vi "Plate Tank 2.vi"() -> ()   [LabVIEW 2019]
uses:
  <vilib>/NI/Current Value Table/Type Defs/Single Tag.ctl
  <vilib>/NI/Current Value Table/Type Defs/Data Types.ctl
  <vilib>/Utility/sysdir.llb/System Directory Type.ctl
  <vilib>/NI/STM/TCP/Read Meta Data (TCP Ref).vi
  <vilib>/NI/STM/TCP/Get Connection Reference (TCP).vi
  <vilib>/NI/AMC/Read Termination Message.vi
  <vilib>/NI/AMC/Create Single Message.vi
  <vilib>/NI/AMC/Update Message Routing Info.vi
  <vilib>/NI/STM/TCP/Read Meta Data (TCP Clst).vi
  <vilib>/NI/AMC/Send Message.vi
  <vilib>/NI/AMC/Globals.vi
  <userlib>/_OpenG.lib/comparison/comparison.llb/I32 Changed__ogtk.vi
  <vilib>/NI/STM/TCP/Write Message (TCP).vi
  <vilib>/NI/AMC/AMC.lvlib
  <vilib>/NI/STM/NI STM.lvlib
  <vilib>/NI/Current Value Table/Current Value Table.lvlib
panel:
  in  "Settings Button":bool
  out "Loaded Recipe":string
  in  "Load A Recipe":bool
  in  "Save this Recipe":bool
  out "Right Time":dbl format="%.1f"
  out "Left Time":dbl format="%.1f"
  out "Total Amp*min R":dbl format="%.1f"
  out "Total Amp*min L":dbl format="%.1f"
  in  "Reverse Current Multiplier":dbl=3.0 min=0.1 max=100.0 step=0.01 format="%.2g"
  in  "Rectifer Settings":i32(listbox)
  in  "Tab Control 3":enum32{"Standard", "Eng"}(tab)
  out "Left Anode Amp-min":dbl(slide) scale=0.0..254.0
  out "Right Anode Amp-min":dbl(slide) scale=0.0..135.0
  out "Left Anode Actual Current":dbl(knob) scale=0.0..150.0
  out "Right Anode Actual Current":dbl(knob) scale=0.0..150.0
  out "Current Step":i32
  out "Output Voltage":cluster{dbl, dbl}(graph)
  in  "MO":string
  in  "Tab Control 2":enum32{"Plating Cell Status", "ENG"}(tab)
  out "Supply Flow":dbl(knob) scale=0.0..65.0 scale format="%#.2g"
  out "Suck Pump":bool
  out "Suck Pump Flow":dbl format="%#_4g"
  out "SuckPipe":bool
  out "Plating Cell Liquid Level":dbl(slide) scale=0.0..75.0
  out "Cell Temperature":dbl(slide) scale=0.0..60.0
  in  "Cell T Last Hr":bool
  in  "Tab Control":enum32{"Main Pump", "Suck Pump"}(tab)
  out "Amps":dbl format="%#.2g"
  out "Volts":dbl format="%#.1f"
  out "VFD T":dbl format="%#.2g"
  out "RPM":dbl format="%#.0f"
  out "Fault Code":dbl format="%#.2g"
  out "Freq":dbl format="%#.2g"
  out "SP1 Amps":dbl caption="Amps" format="%#.2g"
  out "SP1 Volts":dbl caption="Volts" format="%#.1g"
  out "SP1 RPM":dbl caption="RPM" format="%#.2g"
  out "SP1 VFD T":dbl caption="VFD T" format="%#.2g"
  out "SP1 Fault Code":dbl caption="Fault Code" format="%#.2g"
  out "SP1 Freq":dbl caption="Freq" format="%#.2g"
  out "Flow 1":dbl format="%#_4g"
  out "Flow 2":dbl format="%#_4g"
  out "Flow 3":dbl format="%#_4g"
  out "Flow 4":dbl format="%#_4g"
  out "Flow Controller":dbl(knob) scale=0.0..100.0
  out "E Stop":bool
  out "Run Enabled?":bool
  in  "Full Drain Plating Cell":bool
  out "Rack Motion":bool
  out "Right Eductor Motion":bool
  out "Left Eductor Motion":bool
  out "Right Output On":bool
  in  "Enable Rack Motion":bool
  in  "Rack RPM":dbl(knob) min=0.0 max=11.0 step=0.125 scale=0.0..11.0
  out "Left Output On":bool
  in  "Start Cycle":bool
  in  "Cancel Cycle":bool
  out "BasTankTee":bool
  out "SuckPipe 2":bool
  out "Main Pump":bool
  in  "Enable Eductor Motion":bool
  in  "Eductor RPM":dbl(knob) min=0.0 max=11.0 step=0.125 scale=0.0..11.0
  in  "Supply Pressure (kPa)":dbl(knob)=50.0 min=50.0 max=200.0 step=5.0 scale=50.0..200.0
  in  "Total Inflow (L/min)":dbl(knob)=40.0 min=25.0 max=50.0 step=1.0 scale=25.0..50.0
  in  "Suck Pump fraction of inflow":dbl(knob)=5.0 min=5.0 max=90.0 step=1.0 scale=0.0..90.0
  out "Sump Level":dbl(slide) scale=0.0..1000.0
  out "Supply Pressure":dbl(knob) scale=0.0..200.0
  in  "Enable Suck Pump":bool
  in  "Enable Plating Cell":bool
  in  "Machine":bool
  in  "Basement 4":bool
  in  "Dryer":bool
  in  "Rinse 4":bool
  in  "Rinse 3":bool
  in  "Rinse 2":bool
  in  "Basement 3":bool
  in  "Basement 2":bool
  in  "Basement 1":bool
  in  "Plater 6":bool
  in  "Plater 5":bool
  in  "Plater 4":bool
  in  "Plater 3":bool
  in  "Plater 2":bool
  in  "Plater 1":bool
  in  "Predip":bool
  in  "Rinse 1":bool
  in  "Cleaner":bool
  in  "Etch":bool
  out "status":string
  # "Module Selection"
  # "Rectifier Settings"
  # "Fluid Flow Control"
  # "Rectifier Control"
  # "Rectifier Output"
  # "Motion starts when rectifiers cycle"
  # "Note: RPM settings shared with tank 1"
  # "kPa"
  # "Output"
  # "cm"
  # "°C"
  # "cm"
  # "L/min"
  # "L/min"
  # "L/min"
  # "L/min"
  # "L/min"
  # "L/min"
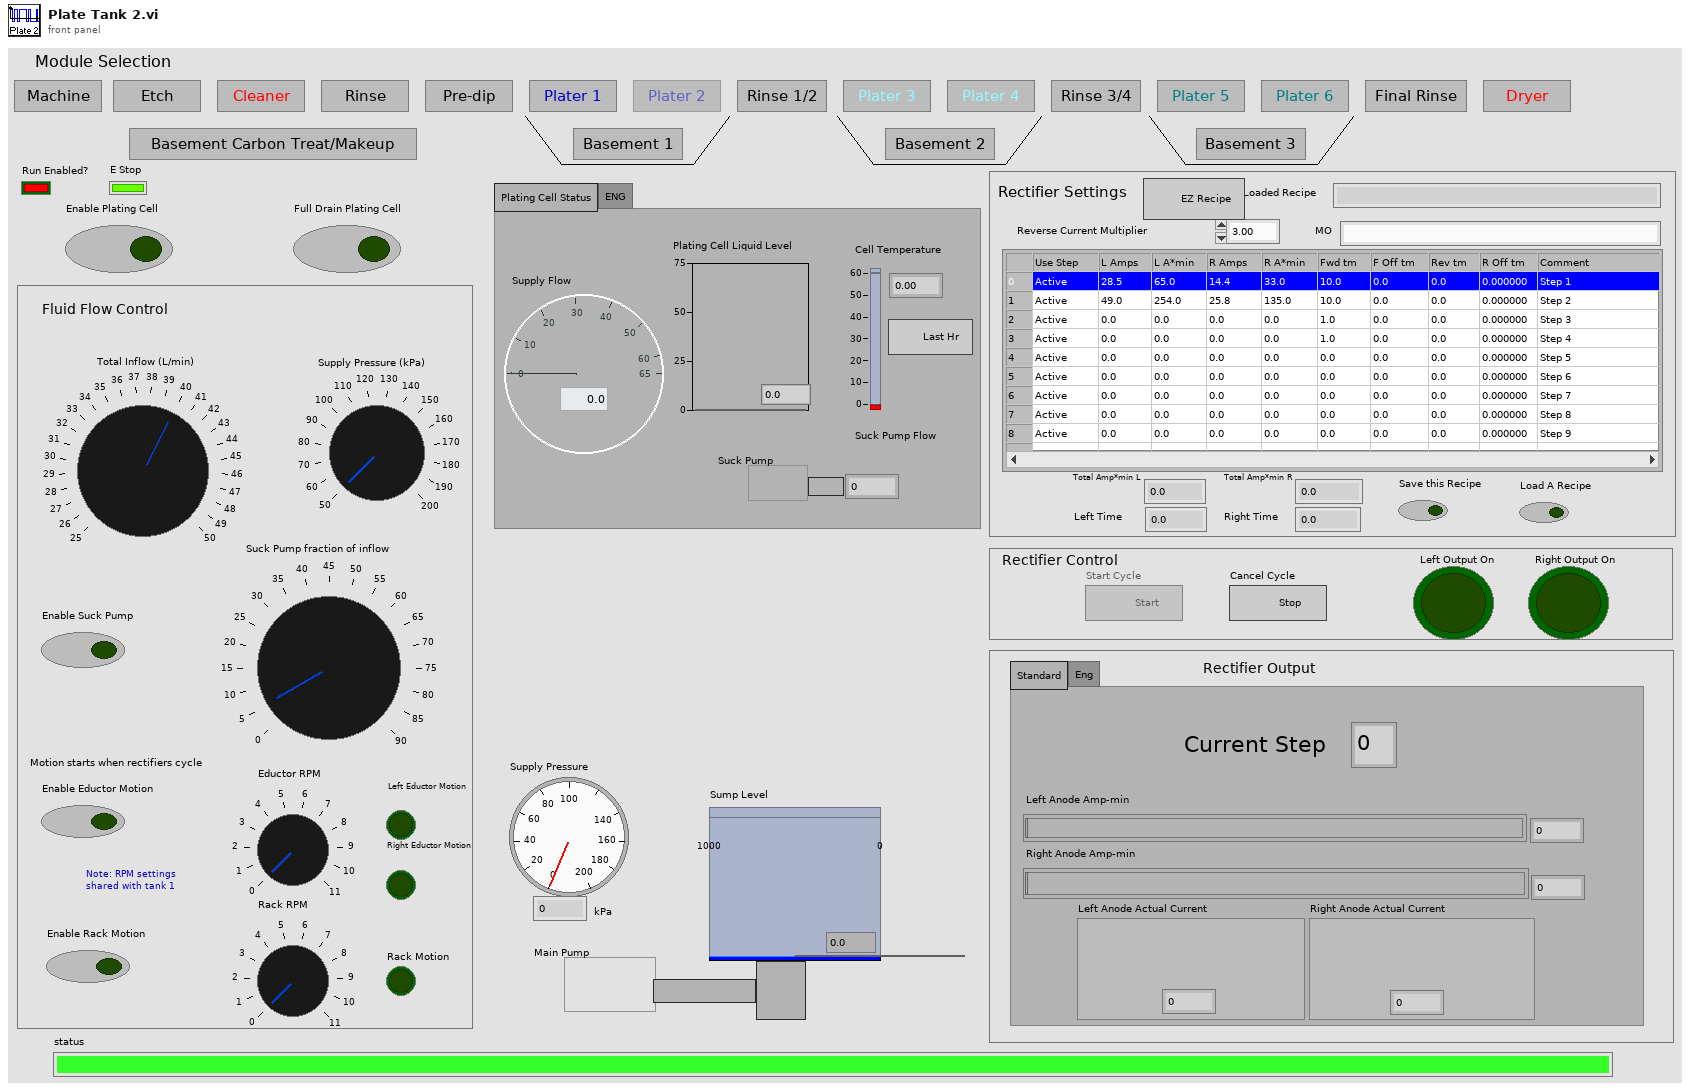
[diagram p1: front panel]
types:
  T1 = typedef "Current Value Table.lvlib/Single Tag.ctl" = cluster{"Data Type":T2, "Name":string, "Value":string, "Description":string}
  T2 = typedef "Current Value Table.lvlib/Data Types.ctl" = enum16{"Double", "Single", "I64", "I32", "I16", "I8", "U64", "U32", "U16", "U8", "String", "Boolean", "Array of U8", "Array of U16", "Array of U32", "Array of U64", "Array of I64", "Array of I32", "Array of I16", "Array of I8", "Array of Double", "Array of Single", "Array of Boolean", "Array of String"}
  T3 = typedef "NI STM.lvlib/TCP Connection Info.ctl" = cluster{"connection ID":refnum<k5>, "meta data":T4[]}
  T4 = typedef "NI STM.lvlib/MetaDataElement.ctl" = string
  T5 = typedef "AMC.lvlib/Message Queue.ctl" = refnum<queue>
  T6 = enum8{"Enabled", "Disabled", "Disabled and Grayed Out"}
  T7 = typedef "System Directory Type.ctl" = i32
  T8 = cluster{"Shift":bool, "Ctrl":bool, "Alt":bool, "Cmd":bool, "Opt":bool}
  T9 = typedef "LVPoint32TypeDef.ctl" = cluster{"Horizontal":i32, "Vertical":i32}
  T10 = typedef "LVRowAndColumnTypeDef.ctl" = cluster{"Row":i32, "Column":i32}
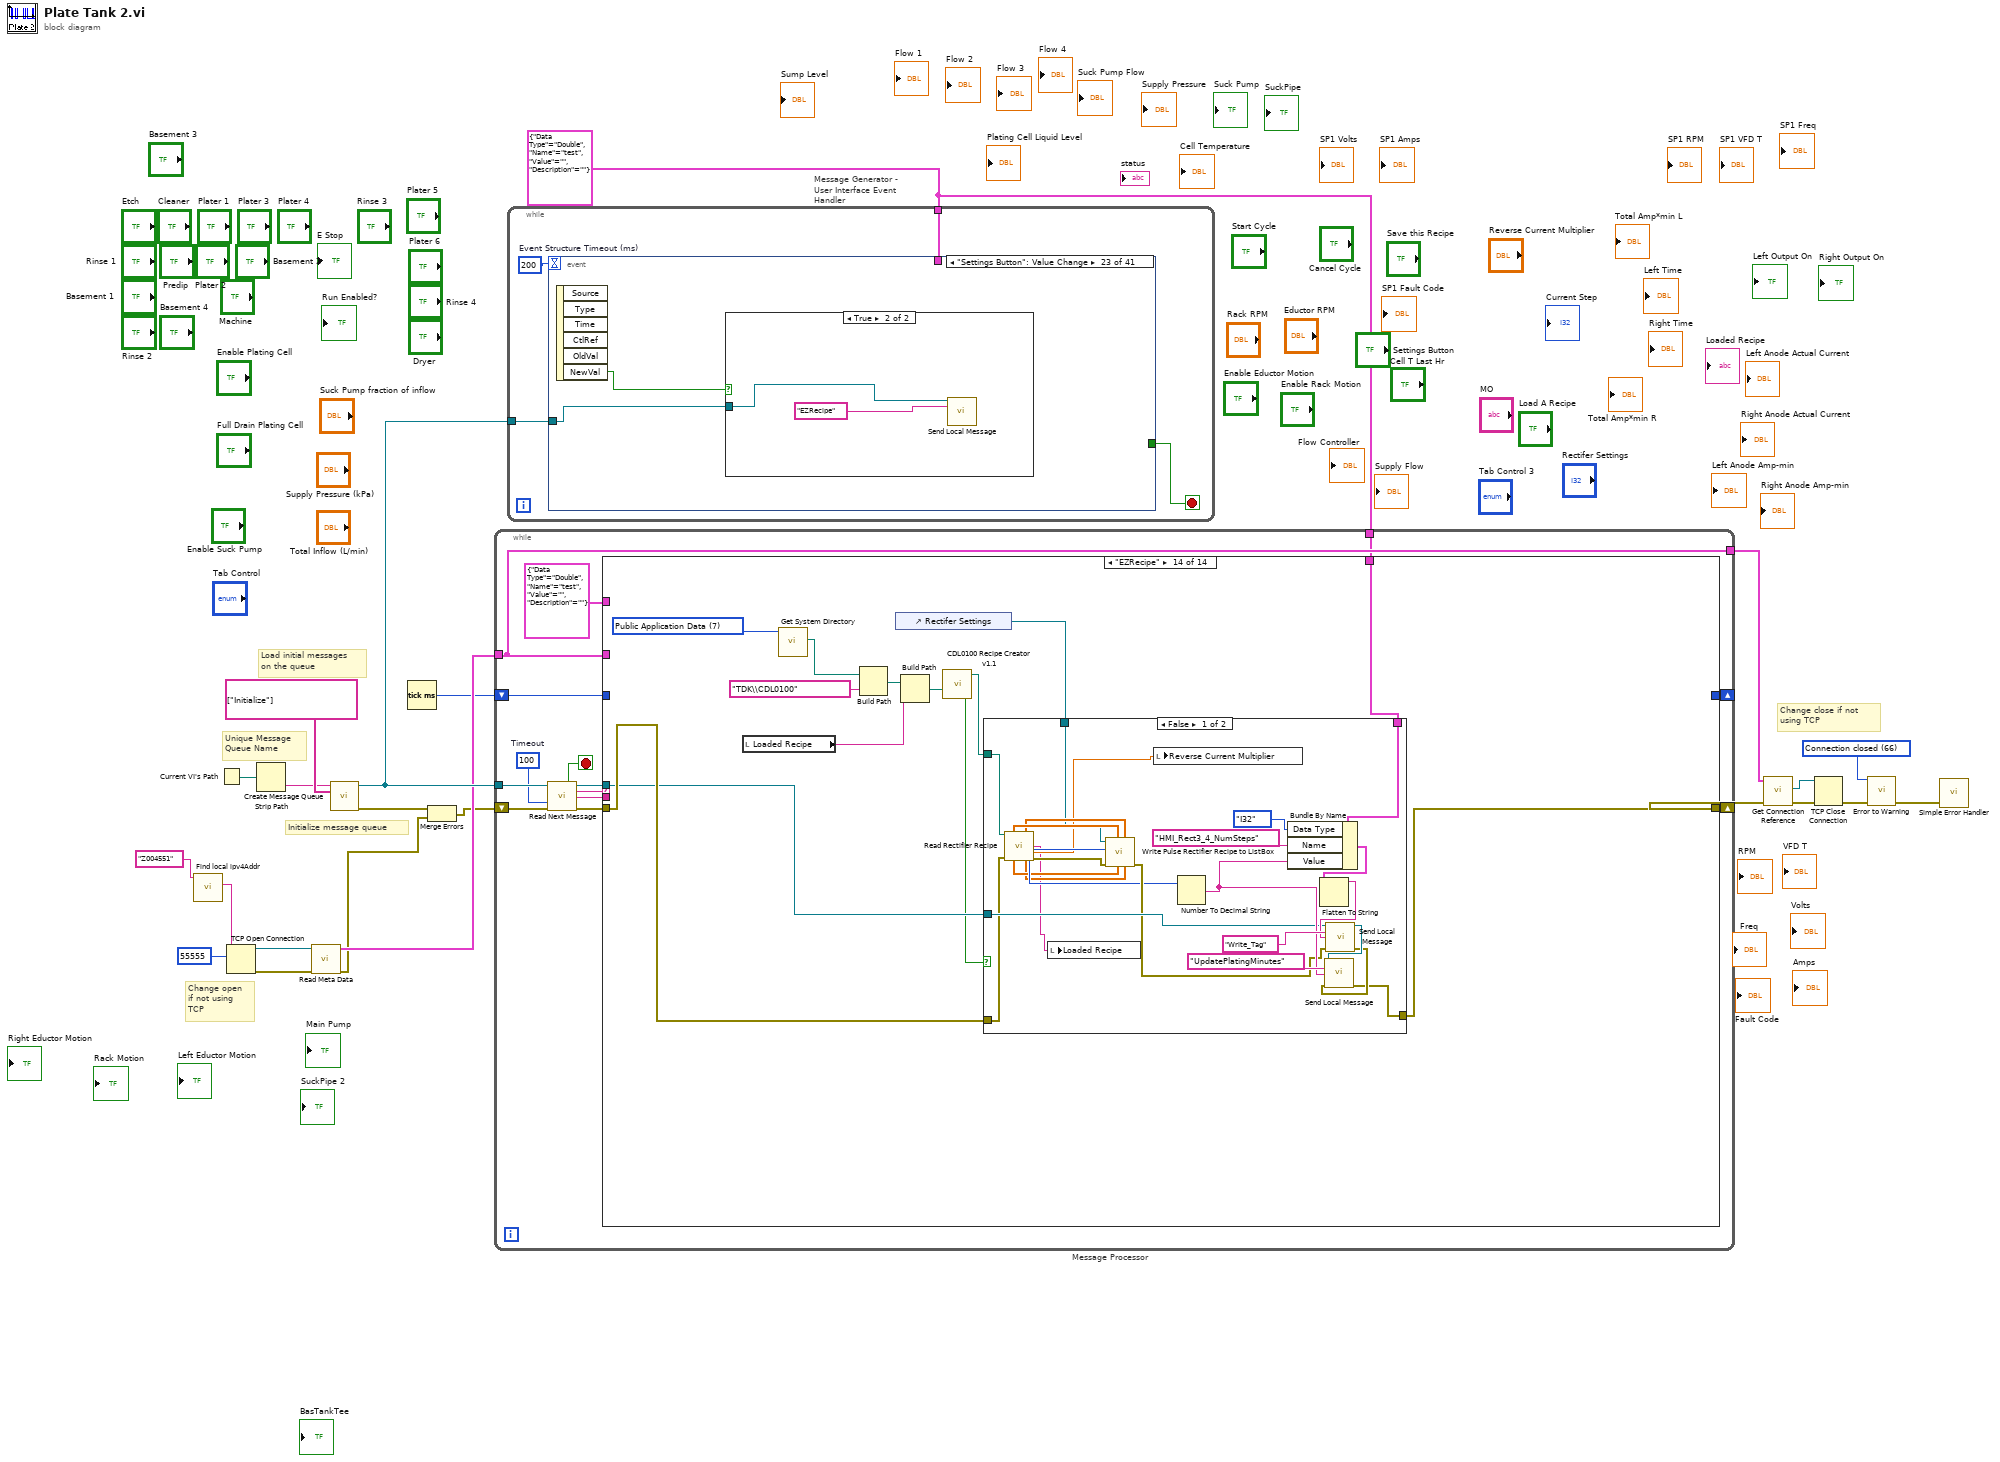
[diagram p0: block diagram]
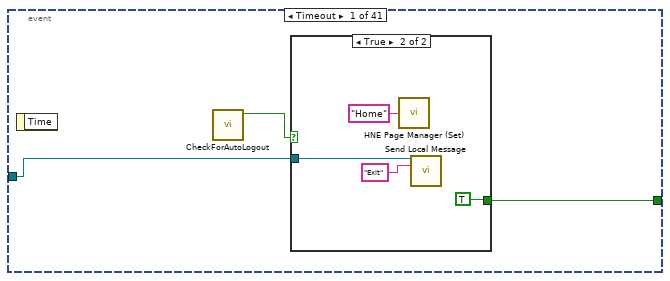
[diagram p2: hidden frame]
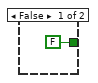
[diagram p3: hidden frame]
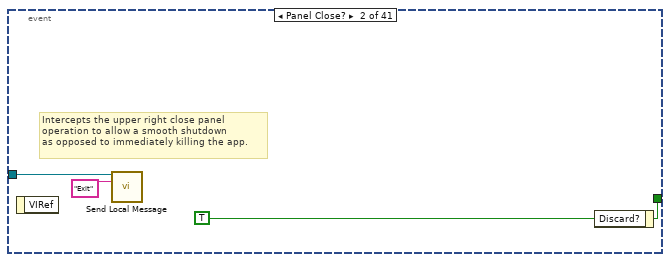
[diagram p4: hidden frame]
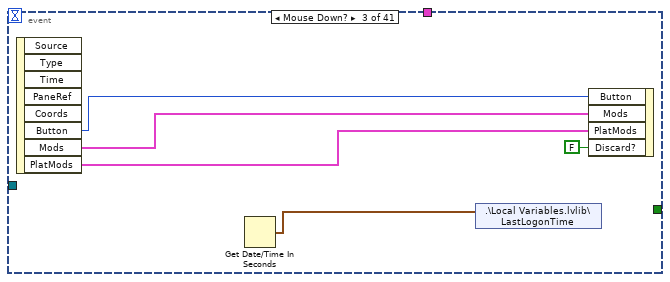
[diagram p5: hidden frame]
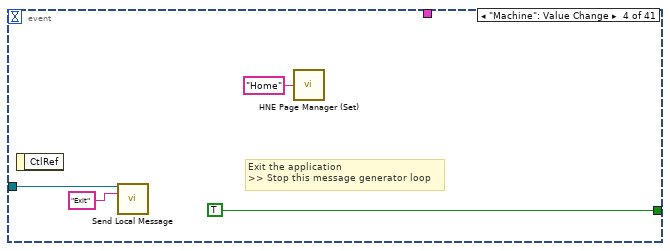
[diagram p6: hidden frame]
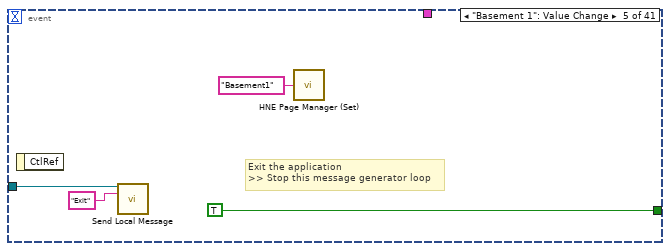
[diagram p7: hidden frame]
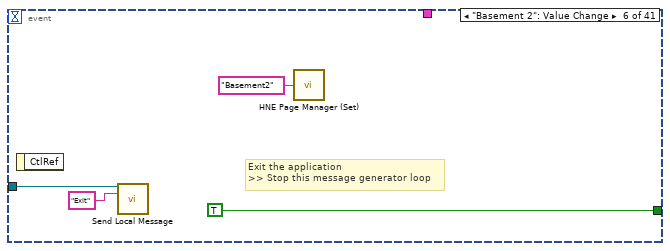
[diagram p8: hidden frame]
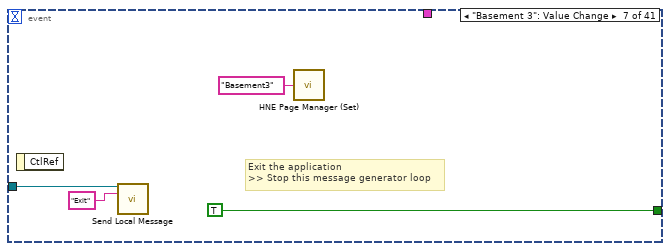
[diagram p9: hidden frame]
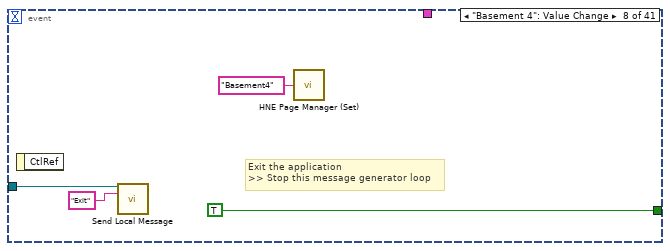
[diagram p10: hidden frame]
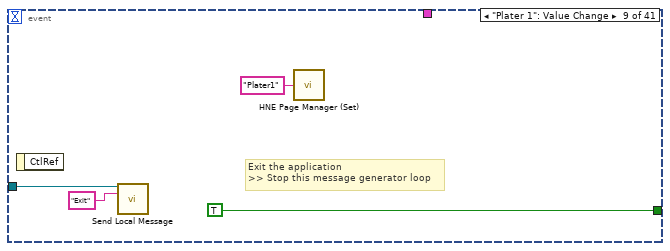
[diagram p11: hidden frame]
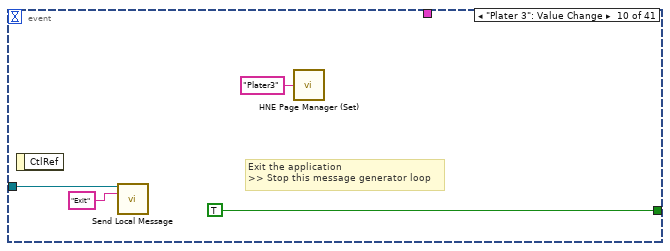
[diagram p12: hidden frame]
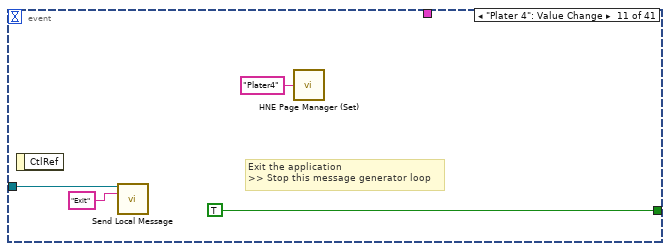
[diagram p13: hidden frame]
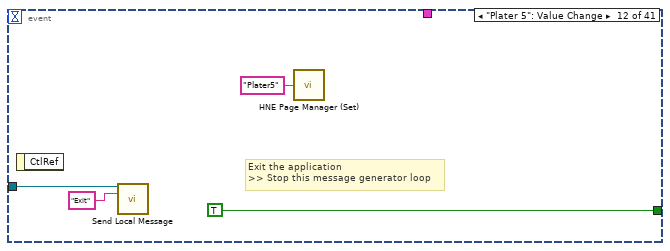
[diagram p14: hidden frame]
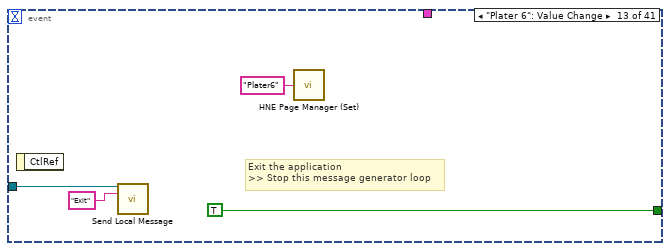
[diagram p15: hidden frame]
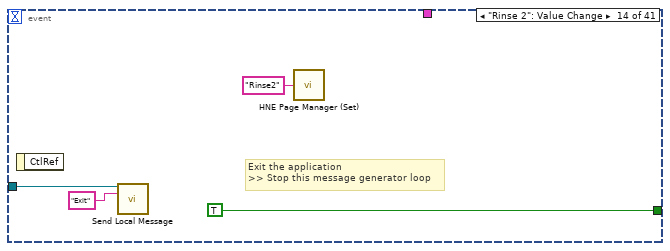
[diagram p16: hidden frame]
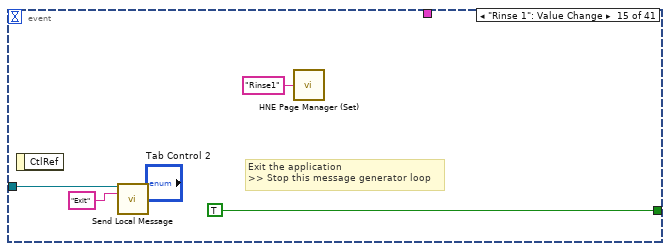
[diagram p17: hidden frame]
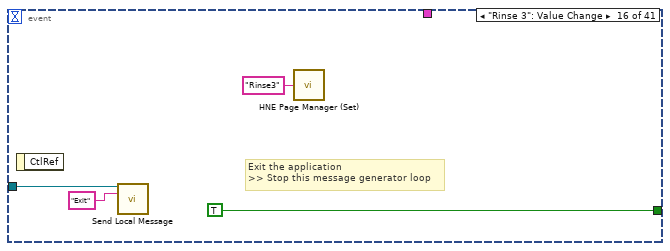
[diagram p18: hidden frame]
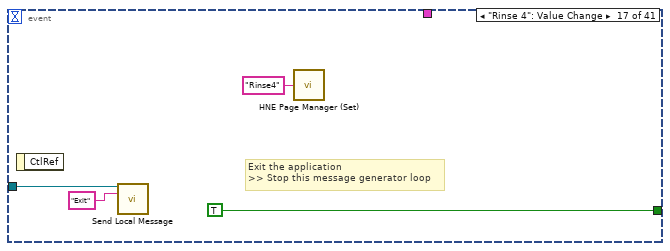
[diagram p19: hidden frame]
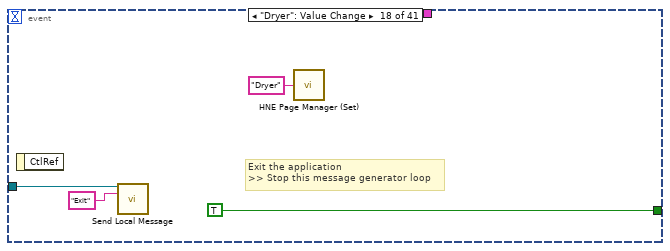
[diagram p20: hidden frame]
diagram:
  w1 = T1 {"Data Type"=enum."Double", "Name"="test", "Value"="", "Description"=""} ("Tag")
  w13 = 66 items=["No Error", "Argument Error", "Memory Full", "Out of Zone", "End of File", "File Already Open", "Generic File IO Error", "File Not Found", "File Permission Error", "Disk Full", "Duplicate Path", "Too Many Files Open", "Not Enabled", "Resource File Not Found", "Cannot Add Resource", "Resource Not Found", "Image Not Found", "Image Memory Error", "Pen Does Not Exist", "Config Bad Type", "Config Token Not Found", "Config Parse Error", "Config Memory Error", "Bad External Code Format", "Bad External Code Offset", "External Code Not Present", "Null Window", "Destroy Window Mixup", "Null Menu", "Print Aborted", "Bad Print Record", "Print Driver Error", "Windows Error During Print", "Memory Error During Print", "Print Dialog Error", "Generic Print Error", "Invalid Device Refnum", "Device Not Found", "Device Parameter Error", "Device Unit Error", "Can't Open Device", "Device Call Aborted", "Generic Error", "Cancelled By User", "Object ID Too Low", "Object ID Too High", "Object Not In Heap", "Unknown Heap", "Bad DefProc ID", "DefProc Not In Table", "Message Out Of Range", "Null Method", "Unknown Message", "Manager Call Not Supported", "Bad address", "Connection In progress", "Connection timed out", "Connection is already in progress", "Network attribute not supported", "Network error", "Address in use", "System out of memory", "Connection aborted", "Connection refused", "Connection is not connected", "Connection is already connected", "Connection closed", "Initialize error (interapplication manager)", "Bad occurrence", "Wait on unbound occurrence handler", "Occurrence queue overflow", "Bad path", "Semaphore not signaled", "Unrecognized type (interapplication manager)"] ("1st Error to Convert")
  # "Change close if not using TCP"
  # "Change open if not using TCP"
  # "Initialize message queue"
  # "Unique Message\nQueue Name"
  # "Load initial messages\non the queue"
  n1 = call "Find local ipv4Addr.vi"("MachineToFind"="Z004551" ("Target IP Address")) -> ("name"=w5:string)  [unwired: 9 in, 1 out]
  n2 = Current VI's Path() -> (path=w19:path)
  n3 = TCP Open Connection(address=w5, remote port or service name=u16 55555 ("remote port")) -> (connection ID=w17:refnum<k5>, error out=w16:errorcluster)  [unwired: 1 in, 2 out]
  n4 = Strip Path(path=w19) -> (name=w21:string)  [unwired: 1 out]
  n5 = call-poly <vilib>:"Read Meta Data.vi"("error in"=w16, "connection ID"=w17) -> ("error out"=w3:errorcluster, "connection info out"=w15:T3)  [unwired: 7 in, 1 out]
  n6 = call <vilib>:"Create Message Queue.vi"("message queue name"=w21, "initial message names"=string[] ["Initialize"]) -> ("message queue out"=w20:T5, "error out"=w4:errorcluster)  [unwired: 12 in]
  n7 = Tick Count (ms)() -> (millisecond timer value=w7:u32)
  n8 = Merge Errors(w4, w3) -> (w2:errorcluster)
  n9 = while "Message Processor" {
    shift-left: w2 -> [w32]
    shift-right: [w36] -> w8
    tunnel: w20 -> [w33]
    tunnel: w15 -> [w27]
    tunnel: [w27] -> w9
    shift-right: [w24] -> _
    shift-left: w7 -> [w25]
    tunnel: w1 -> [w23]
    stop <- w35 stop-if-true
    w28 = 100  # Timeout
    n10 = call <vilib>:"Read Next Message.vi"("message queue in"=w33, "timeout (1 ms)"=w28, "error in"=w32) -> ("exit process?"=w35:bool, "message queue out"=w34:T5, "message name"=w30:string, "message value"=w29:string, "error out"=w31:errorcluster)  [unwired: 5 in, 3 out]
    n11 = case shown="\"EZRecipe\"" w30 {
      selector: w30 -> [_ _ w110 _ _ _ _ _ _ _ _ _ _ _]
      tunnel: w34 -> [_ _ _ _ _ _ w259 _ _ _ w283 _ w304 w340]
      tunnel: w31 -> [w37 w49 w111 w112 w114 w116 w260 w262 w266 w269 w282 w297 w308 w341]
      tunnel: [w37 w49 w111 errorcluster {"status"=FALSE, "code"=0, "source"=""} ("error out") w114 w116 w258 w262 w265 w269 w281 w295 w301 w336] -> w36
      tunnel: w29 -> [_ _ _ _ _ _ _ _ w264 w271 w277 _ _ _]
      tunnel: w27 -> [_ _ _ _ _ _ _ _ w267 _ _ _ _ _]
      tunnel: T1 {"Data Type"=enum."Double", "Name"="test", "Value"="", "Description"=""} ("Tag") -> [_ _ _ _ _ _ _ _ _ _ _ _ _ _]
      tunnel: w25 -> [_ w44 _ _ _ w115 _ _ w263 w270 w280 w299 w309 _]
      tunnel: [_ w45 _ _ _ w115 _ _ w263 w270 w280 w299 w309 _] -> w24
      tunnel: w23 -> [_ _ _ _ _ _ _ _ _ _ _ _ w303 w337]
      frame "---------- Framework Operations ----------" {
        # "Dummy case to add a seperator in the Case Structure menu"
      }
      frame "", "Idle" {
        n12 = stacked-sequence {
          frame #0 {
            n13 = shared-variable-read(refnum<k21> "ni.var.psp://z004551/CDL0100 ReadTags/Tnk2_Can_Plate" ("shared variable refnum in"), FALSE) -> (w64:bool)  [unwired: 1 in, 3 out]
            n14 = shared-variable-read(refnum<k21> "ni.var.psp://z004551/CDL0100 ReadWriteTags/HMI_Tank2_Drain" ("shared variable refnum in"), FALSE) -> (w52:bool)  [unwired: 1 in, 3 out]
            n15 = control-ref of="Start Cycle"() -> (w66:refnum<vi>)
            n16 = shared-variable-read(refnum<k21> "ni.var.psp://z004551/CDL0100 ReadWriteTags/HMI_Enable_BTnk1_Pump" ("shared variable refnum in"), FALSE) -> (w58:bool)  [unwired: 1 in, 3 out]
            n17 = shared-variable-read(refnum<k21> "ni.var.psp://z004551/CDL0100 ReadWriteTags/HMI_Tank2_Enable" ("shared variable refnum in"), FALSE) -> (w59:bool)  [unwired: 1 in, 3 out]
            n18 = case shown="False" w64 {
              tunnel: [T6."Disabled and Grayed Out" ("Disabled") T6."Enabled" ("Disabled")] -> w65
              frame False {
              }
              frame True {
              }
            }
            n19 = Or(x=w59, y=w58) -> (x .or. y?=w57:bool)
            n20 = case shown="True" w52 {
              tunnel: [T6."Enabled" ("Disabled") T6."Disabled and Grayed Out" ("Disabled")] -> w51
              frame False {
              }
              frame True {
              }
            }
            n21 = case shown="True" w57 {
              tunnel: [T6."Enabled" ("Disabled") T6."Disabled and Grayed Out" ("Disabled")] -> w56
              frame False {
              }
              frame True {
              }
            }
            n22 = control-ref of="Full Drain Plating Cell"() -> (w55:refnum<vi>)
            n23 = control-ref of="Enable Plating Cell"() -> (w50:refnum<vi>)
            n24 = property class="Bool (strict)"(reference=w66, "DisabledEnum"=w65) -> ()  [unwired: 1 in, 2 out]
            n25 = property class="Bool (strict)"(reference=w50, "DisabledEnum"=w51) -> ()  [unwired: 1 in, 2 out]
            n26 = property class="Bool (strict)"(reference=w55, "DisabledEnum"=w56) -> ()  [unwired: 1 in, 2 out]
          }
          frame #1 {
            n27 = shared-variable-read(refnum<k21> "ni.var.psp://z004551/CDL0100 ReadTags/Rect3_4_CurrRecpStp" ("shared variable refnum in"), 0) -> (w75:i32)  [unwired: 1 in, 3 out]
            n28 = call-poly <userlib>:"Data Changed__ogtk.vi"("I32"=w75) -> ("Changed"=w76:bool)
            n29 = case shown="True" w76 {
              tunnel: w75 -> [_ w80]
              frame False {
              }
              frame True {
                w85 = 0.0 ("Scale.Range:Minimum")
                n30 = control-ref of="Right Anode Amp-min"() -> (w81:refnum<vi>)
                n31 = shared-variable-read(refnum<k21> "ni.var.psp://z004551/CDL0100 ReadWriteTags/HMI_Rect3_4_NumSteps" ("shared variable refnum in"), 0) -> (w79:i32)  [unwired: 1 in, 3 out]
                n32 = Less?(x=w80, y=w79) -> (x < y?=w93:bool)
                n33 = case shown="False" w93 {
                  tunnel: w80 -> [w97 w98]
                  tunnel: [w96 w98] -> w92
                  frame False {
                    n34 = Decrement(x=w97) -> (x-1=w96:i32)
                  }
                  frame True {
                  }
                }
                n35 = shared-variable-read(refnum<k21> "ni.var.psp://z004551/CDL0100 ReadWriteTags/HMI_Rct4_AMin_SetPnts" ("shared variable refnum in"), dbl[] []) -> (w86:dbl[])  [unwired: 1 in, 3 out]
                n36 = control-ref of="Left Anode Amp-min"() -> (w82:refnum<vi>)
                n37 = Index Array(array=w86, index=w92) -> (element=w83:dbl)
                n38 = shared-variable-read(refnum<k21> "ni.var.psp://z004551/CDL0100 ReadWriteTags/HMI_Rct3_AMin_SetPnts" ("shared variable refnum in"), dbl[] []) -> (w89:dbl[])  [unwired: 1 in, 3 out]
                n39 = Index Array(array=w89, index=w92) -> (element=w84:dbl)
                n40 = property class="Slide (strict)"(reference=w82, "Scale.Maximum"=w84, "Scale.Minimum"=w85) -> ()  [unwired: 1 in, 2 out]
                n41 = property class="Slide (strict)"(reference=w81, "Scale.Maximum"=w83, "Scale.Minimum"=w85) -> ()  [unwired: 1 in, 2 out]
              }
            }
          }
        }
        n42 = local read "Left Output On"() -> (w41:bool)
        n43 = local read "Right Output On"() -> (w42:bool)
        n44 = Tick Count (ms)() -> (millisecond timer value=w43:u32)
        n45 = Subtract(x=w43, y=w44) -> (x-y=w46:u32)
        n46 = Or(x=w41, y=w42) -> (x .or. y?=w40:bool)
        n47 = Greater?(x=w46, y=u32 500) -> (0:w39:bool)
        n48 = And(x=w40, y=w39) -> (x .and. y?=w38:bool)
        n49 = case shown="True" w38 {
          tunnel: w43 -> [_ w100]
          tunnel: [w99 w100] -> w45
          tunnel: w44 -> [w99 _]
          frame False {
          }
          frame True {
            n50 = shared-variable-read(refnum<k21> "ni.var.psp://z004551/CDL0100 ReadTags/Rect3_ActlVolts" ("shared variable refnum in"), 0.0) -> (w103:dbl)  [unwired: 1 in, 3 out]
            n51 = shared-variable-read(refnum<k21> "ni.var.psp://z004551/CDL0100 ReadTags/Rect4_ActlVolts" ("shared variable refnum in"), 0.0) -> (w102:dbl)  [unwired: 1 in, 3 out]
            n52 = Bundle(w103, w102) -> (→"Output Voltage":cluster{dbl, dbl})  [unwired: 1 in]
          }
        }
        n53 = control-ref of="status"() -> (w48:refnum<vi>)
        n54 = call <userlib>:"TAE Format Alarm Ticker.vi"("Alarm Ticker Ref"=w48) -> ()  [unwired: 15 in]
      }
      frame "Missing Message Handler", Default {
        # "Call this case if a message is received that is not handled \nby any other case. Typically this is a programming error\nas a result of a typo or unhandled message/missing message handler."
        n55 = Format Into String(format string="DevError: Missing message handler for '%s\" message." ("message"), w110) -> (resulting string=w108:string)  [unwired: 2 in, 1 out]
        n56 = One Button Dialog(message=w108) -> ()  [unwired: 2 out]
      }
      frame "Error" {
        # "General Error Case - this case is called if an error is passed using the error cluster below. Typically most new errors should be handed in each individual case and not passed in the rror cluster. If necessary a custom error handler case should be added and called from other cases."
        n57 = call <vilib>:"Simple Error Handler.vi"("error in (no error)"=w112) -> ()  [unwired: 1 in, 8 out]
      }
      frame "---------- Generic Operations ----------" {
        # "Dummy case to add a seperator in the Case Structure menu"
      }
      frame "Initialize" {
        n58 = stacked-sequence {
          seq-local: [_ _ w155 _ _ _] -> [_ _ _ _ w193 w246]
          seq-local: [_ _ w156 _ _ _] -> [_ _ _ _ w192 _]
          seq-local: [_ _ w151 _ _ _] -> [_ _ _ _ w191 w237]
          seq-local: [_ _ _ w175 _ _] -> [_ _ _ _ w190 _]
          seq-local: [_ _ _ w174 _ _] -> [_ _ _ _ w188 _]
          seq-local: [_ _ _ w173 _ _] -> [_ _ _ _ w187 _]
          seq-local: [_ _ _ w172 _ _] -> [_ _ _ _ w186 _]
          seq-local: [_ w134 _ _ _ _] -> [_ _ w149 _ w184 w236]
          frame #0 {
            n59 = shared-variable-read(refnum<k21> "ni.var.psp://z004551/CDL0100 ReadWriteTags/HMI_TNK2_SuckPmpFrac_Setpoint" ("shared variable refnum in"), 0.0) -> (w119:dbl)  [unwired: 1 in, 3 out]
            n60 = shared-variable-read(refnum<k21> "ni.var.psp://z004551/CDL0100 ReadWriteTags/HMI_Tnk2_Enable_SuckPump" ("shared variable refnum in"), FALSE) -> (w122:bool)  [unwired: 1 in, 3 out]
            n61 = shared-variable-read(refnum<k21> "ni.var.psp://z004551/CDL0100 ReadWriteTags/HMI_Tnk1_Rack_RPM" ("shared variable refnum in"), 0.0) -> (w133:dbl)  [unwired: 1 in, 3 out]
            n62 = shared-variable-read(refnum<k21> "ni.var.psp://z004551/CDL0100 ReadWriteTags/HMI_Tank2_Rack_Motor_Run" ("shared variable refnum in"), FALSE) -> (w132:bool)  [unwired: 1 in, 3 out]
            n63 = shared-variable-read(refnum<k21> "ni.var.psp://z004551/CDL0100 ReadWriteTags/HMI_TNK2_Flow_Setpoint" ("shared variable refnum in"), 0.0) -> (w131:dbl)  [unwired: 1 in, 3 out]
            n64 = Multiply(x=w119, y=100.0) -> (x*y=w117:dbl)
            n65 = local write "Enable Suck Pump"(w122) -> ()
            n66 = local write "Rack RPM"(w133) -> ()
            n67 = local write "Enable Rack Motion"(w132) -> ()
            n68 = local write "Total Inflow (L/min)"(w131) -> ()
            n69 = local write "Suck Pump fraction of inflow"(w117) -> ()
          }
          frame #1 {
            n70 = shared-variable-read(refnum<k21> "ni.var.psp://z004551/CDL0100 ReadWriteTags/HMI_Tank2_Drain" ("shared variable refnum in"), FALSE) -> (w137:bool)  [unwired: 1 in, 3 out]
            n71 = shared-variable-read(refnum<k21> "ni.var.psp://z004551/CDL0100 ReadWriteTags/HMI_Tnk1_Eductor_RPM" ("shared variable refnum in"), 0.0) -> (w145:dbl)  [unwired: 1 in, 3 out]
            n72 = shared-variable-read(refnum<k21> "ni.var.psp://z004551/CDL0100 ReadWriteTags/HMI_Rect3_4_NumSteps" ("shared variable refnum in"), 0) -> (w134:i32)  [unwired: 1 in, 3 out]
            n73 = shared-variable-read(refnum<k21> "ni.var.psp://z004551/CDL0100 ReadWriteTags/HMI_Tank2_Enable" ("shared variable refnum in"), FALSE) -> (w144:bool)  [unwired: 1 in, 3 out]
            n74 = local write "Full Drain Plating Cell"(w137) -> ()
            n75 = shared-variable-read(refnum<k21> "ni.var.psp://z004551/CDL0100 ReadWriteTags/HMI_Tank2_Eductor_Motors_Run" ("shared variable refnum in"), FALSE) -> (w148:bool)  [unwired: 1 in, 3 out]
            n76 = local write "Enable Plating Cell"(w144) -> ()
            n77 = local write "Eductor RPM"(w145) -> ()
            n78 = local write "Enable Eductor Motion"(w148) -> ()
          }
          frame #2 {
            n79 = shared-variable-read(refnum<k21> "ni.var.psp://z004551/CDL0100 ReadWriteTags/HMI_BAS_TNK1_P_Setpoint" ("shared variable refnum in"), 0.0) -> (w163:dbl)  [unwired: 1 in, 3 out]
            n80 = local write "Supply Pressure (kPa)"(w163) -> ()
            n81 = shared-variable-read(refnum<k21> "ni.var.psp://z004551/CDL0100 ReadWriteTags/HMI_Rct3_AMin_SetPnts" ("shared variable refnum in"), dbl[] []) -> (w155:dbl[])  [unwired: 1 in, 3 out]
            n82 = shared-variable-read(refnum<k21> "ni.var.psp://z004551/CDL0100 ReadWriteTags/HMI_Rct4_AFwd_SetPnts" ("shared variable refnum in"), dbl[] []) -> (w156:dbl[])  [unwired: 1 in, 3 out]
            n83 = shared-variable-read(refnum<k21> "ni.var.psp://z004551/CDL0100 ReadWriteTags/HMI_Rct4_AMin_SetPnts" ("shared variable refnum in"), dbl[] []) -> (w151:dbl[])  [unwired: 1 in, 3 out]
            n84 = for {
              N: w149 -> [_]
              tunnel: w155 -> [w171] mode=indexing
              shift-right: [w169] -> w153
              shift-left: 0.0 -> [w170]
              n85 = Add(x=w171, y=w170) -> (x+y=w169:dbl)
            }
            n86 = for {
              N: w149 -> [_]
              tunnel: w151 -> [w168] mode=indexing
              shift-right: [w166] -> w150
              shift-left: 0.0 -> [w167]
              n87 = Add(x=w168, y=w167) -> (x+y=w166:dbl)
            }
            n88 = local write "Total Amp*min L"(w153) -> ()
            n89 = local write "Total Amp*min R"(w150) -> ()
          }
          frame #3 {
            n90 = shared-variable-read(refnum<k21> "ni.var.psp://z004551/CDL0100 ReadWriteTags/HMI_Rct3_FwdOffTm_SetPnts" ("shared variable refnum in"), dbl[] []) -> (w174:dbl[])  [unwired: 1 in, 3 out]
            n91 = shared-variable-read(refnum<k21> "ni.var.psp://z004551/CDL0100 ReadWriteTags/HMI_Rct3_FwdTm_SetPnts" ("shared variable refnum in"), dbl[] []) -> (w175:dbl[])  [unwired: 1 in, 3 out]
            n92 = shared-variable-read(refnum<k21> "ni.var.psp://z004551/CDL0100 ReadWriteTags/HMI_Rct3_BwdTm_SetPnts" ("shared variable refnum in"), dbl[] []) -> (w173:dbl[])  [unwired: 1 in, 3 out]
            n93 = shared-variable-read(refnum<k21> "ni.var.psp://z004551/CDL0100 ReadWriteTags/HMI_Rct3_BwdOffTm_SetPnts" ("shared variable refnum in"), dbl[] []) -> (w172:dbl[])  [unwired: 1 in, 3 out]
          }
          frame #4 {
            n94 = shared-variable-read(refnum<k21> "ni.var.psp://z004551/CDL0100 ReadWriteTags/HMI_Rct3_AFwd_SetPnts" ("shared variable refnum in"), dbl[] []) -> (w194:dbl[])  [unwired: 1 in, 3 out]
            n95 = for {
              N: 10 -> [_]
              tunnel: w194 -> [w229] mode=indexing
              tunnel: w193 -> [w228] mode=indexing
              tunnel: w192 -> [w227] mode=indexing
              tunnel: w191 -> [w226] mode=indexing
              tunnel: w190 -> [w225] mode=indexing
              tunnel: [w220] -> w189 mode=indexing
              tunnel: w188 -> [w215] mode=indexing
              tunnel: w187 -> [w214] mode=indexing
              tunnel: w186 -> [w213] mode=indexing
              tunnel: [w209] -> w185 mode=indexing
              i -> [w206]
              (unwired) i16 1 ("precision (6)")
              n96 = Number To Fractional String(number=w225, precision (6)=i16 1) -> (F-format string=w216:string)  [unwired: 2 in]
              n97 = Number To Fractional String(number=w226, precision (6)=i16 1) -> (F-format string=w217:string)  [unwired: 2 in]
              n98 = Number To Fractional String(number=w228, precision (6)=i16 1) -> (F-format string=w219:string)  [unwired: 2 in]
              n99 = Number To Fractional String(number=w227, precision (6)=i16 1) -> (F-format string=w218:string)  [unwired: 2 in]
              n100 = Number To Fractional String(number=w229, precision (6)=i16 1) -> (F-format string=w221:string)  [unwired: 2 in]
              n101 = Number To Decimal String(number=w206) -> (decimal integer string=w220:string)  [unwired: 1 in]
              n102 = Number To Fractional String(number=w215, precision (6)=i16 1) -> (F-format string=w212:string)  [unwired: 2 in]
              n103 = Number To Fractional String(number=w214, precision (6)=i16 1) -> (F-format string=w211:string)  [unwired: 2 in]
              n104 = Number To Fractional String(number=w213) -> (F-format string=w210:string)  [unwired: 3 in]
              n105 = Increment(x=w206) -> (x+1=w207:i32)
              n106 = call "Build Text"("d"=w207) -> ("Result"=w208:string)  [unwired: 13 in, 1 out]
              n107 = Build Array("Active", w221, w219, w218, w217, w216, w212, w211, w210, w208) -> (w209:string[])
            }
            n108 = control-ref of="Rectifer Settings"() -> (w197:refnum<vi>)
            n109 = Subtract(x=10, y=w184) -> (x-y=w202:i32)
            n110 = Initialize Array(38, w184) -> (w201:i32[])
            n111 = Initialize Array(37, w202) -> (w200:i32[])
            n112 = Build Array (concatenate)(w201, w200) -> (w196:i32[])
            n113 = property class="MCListbox (strict)"(reference=w197, "ItemSyms"=w196, "RowHdrs[]"=w189, "ItemNames"=w185) -> ()  [unwired: 1 in, 2 out]
          }
          frame #5 {
            n114 = control-ref of="Rectifer Settings"() -> (w254:refnum<vi>)
            n115 = local read "Reverse Current Multiplier"() -> (w252:dbl)
            n116 = property class="MCListbox (strict)"(reference=w254) -> ("ItemNames"=w253:string[][])  [unwired: 1 in, 2 out]
            n117 = shared-variable-read(refnum<k21> "ni.var.psp://z004551/CDL0100 ReadTags/Rect3_4_CurrRecpStp" ("shared variable refnum in"), 0) -> (w235:i32)  [unwired: 1 in, 3 out]
            n118 = shared-variable ".\\Local Variables.lvlib\\PT2_MO"() -> (w249:string)  [unwired: 1 in, 1 out]
            n119 = Less?(x=w235, y=w236) -> (x < y?=w245:bool)
            n120 = case shown="False" w245 {
              tunnel: w235 -> [w256 w257]
              tunnel: [w255 w257] -> w241
              frame False {
                n121 = Decrement(x=w256) -> (x-1=w255:i32)
              }
              frame True {
              }
            }
            n122 = call "Calculate Plating Time.vi"("Num Steps"=w236, "ItemNames"=w253, "Reverse Current Multiplier"=w252) -> ("Right Anode Time"=w250:dbl, "Left Anode Time"=w251:dbl)  [unwired: 7 in]
            n123 = local write "Left Time"(w251) -> ()
            n124 = local write "Right Time"(w250) -> ()
            n125 = local write "MO"(w249) -> ()
            n126 = Index Array(array=w237, index=w241) -> (element=w239:dbl)
            n127 = Index Array(array=w246, index=w241) -> (element=w243:dbl)
            n128 = control-ref of="Left Anode Amp-min"() -> (w244:refnum<vi>)
            n129 = control-ref of="Right Anode Amp-min"() -> (w240:refnum<vi>)
            n130 = property class="Slide (strict)"(reference=w244, "Scale.Maximum"=w243, "Scale.Minimum"=0.0 ("Scale.Range:Minimum")) -> ()  [unwired: 1 in, 2 out]
            n131 = property class="Slide (strict)"(reference=w240, "Scale.Maximum"=w239, "Scale.Minimum"=0.0 ("Scale.Range:Minimum")) -> ()  [unwired: 1 in, 2 out]
          }
        }
      }
      frame "Exit" {
        # "Destroy message queue >> this will halt the UI event handler loop"
        # "Stop the VI\n>> Perform any cleanup tasks in this message case.\n>> Clear display before closing."
        n132 = call <vilib>:"Destroy Message Queue.vi"("message queue in"=w259, "error in"=w260) -> ("error out"=w258:errorcluster)  [unwired: 11 in, 2 out]
        n133 = local write "status"("" ("Status")) -> ()
      }
      frame "---------- Application Operations ----------" {
        # "Dummy case to add a seperator in the Case Structure menu"
      }
      frame "Write_Tag" {
        n134 = call-poly <vilib>:"Write Message.vi"("error in"=w266, "data"=w264, "name"="WriteTag", "connection info in"=w267) -> ("error out"=w265:errorcluster)  [unwired: 6 in, 1 out]
      }
      frame "DisplayLastHr" {
        n135 = call "Trace Variable 1 hour Popup.vi"("Tag"=w271) -> ()  [unwired: 11 in]
      }
      frame "UpdatePlatingMinutes" {
        n136 = Decimal String To Number(string=w277) -> (number=w276:i32)  [unwired: 2 in, 1 out]
        n137 = local read "Reverse Current Multiplier"() -> (w278:dbl)
        n138 = control-ref of="Rectifer Settings"() -> (w279:refnum<vi>)
        n139 = call "Assemble Rectifier Setting Changes for PLC.vi"("Num Steps"=w276, "Rect Number"=3, "error In"=w282, "Reverse Current Multiplier"=w278, "message queue in"=w283, "MulticolumnListbox in"=w279) -> ("Right Anode Mins"=w272:dbl, "Left Anode Mins"=w273:dbl, "Right AmpMin"=w274:dbl, "Left AmpMin"=w275:dbl, "error out"=w281:errorcluster)  [unwired: 1 in]
        n140 = local write "Right Time"(w272) -> ()
        n141 = local write "Total Amp*min R"(w274) -> ()
        n142 = local write "Total Amp*min L"(w275) -> ()
        n143 = local write "Left Time"(w273) -> ()
      }
      frame "Save_Recipe" {
        n144 = local read "Reverse Current Multiplier"() -> (w287:dbl)
        n145 = control-ref of="Rectifer Settings"() -> (w298:refnum<vi>)
        n146 = call "Convert RectifierListData to Arrays.vi"("MulticolumnListbox in"=w298, "error in (no error)"=w297) -> ("Left Amps"=w294:dbl[], "Right Amps"=w293:dbl[], "Left AmpMins"=w292:dbl[], "Right Amp Min"=w291:dbl[], "error out"=w296:errorcluster)  [unwired: 5 in, 4 out]
        n147 = shared-variable-read(refnum<k21> "ni.var.psp://z004551/CDL0100 ReadWriteTags/HMI_Rect3_4_NumSteps" ("shared variable refnum in"), 0) -> (w288:i32)  [unwired: 1 in, 3 out]
        n148 = call "Save Rectifier Recipe.vi"("Rev Mult"=w287, "Right AmpMins"=w291, "Left AmpMins"=w292, "error in"=w296, "Number Steps"=w288, "Right Amps"=w293, "Left Amps"=w294) -> ("error out"=w295:errorcluster, "name"=w285:string, "cancelled"=w286:bool)  [unwired: 2 in]
        n149 = case shown="False" w286 {
          tunnel: w285 -> [w300 _]
          frame False {
            n150 = local write "Loaded Recipe"(w300) -> ()
          }
          frame True {
          }
        }
      }
      frame "Load_A_Recipe" {
        n151 = call "BrowseRecipe.vi"("error in (no error)"=w308) -> ("error out"=w305:errorcluster, "cancelled"=w307:bool, "selected path"=w306:path)  [unwired: 8 in]
        n152 = control-ref of="Rectifer Settings"() -> (w302:refnum<vi>)
        n153 = case shown="False" w307 {
          tunnel: w305 -> [w315 w334]
          tunnel: [w310 w334] -> w301
          tunnel: w304 -> [w325 _]
          tunnel: w303 -> [w324 _]
          tunnel: w306 -> [w314 _]
          tunnel: w302 -> [w313 _]
          frame False {
            n154 = call "Read Rectifier Recipe.vi"("selected path"=w314, "error in"=w315) -> ("Left Amps"=w321:dbl[], "Left AmpMins"=w320:dbl[], "Num Steps"=w319:i32, "name"=w311:string, "Rev Mult"=w312:dbl, "Right Amps"=w318:dbl[], "Right AmpMins"=w317:dbl[], "error out"=w316:errorcluster)  [unwired: 5 in, 1 out]
            n155 = local write "Loaded Recipe"(w311) -> ()
            n156 = call "Write Pulse Rectifier Recipe to ListBox.vi"("Right AmpMins"=w317, "Left AmpMins"=w320, "Right Amps"=w318, "Left Amps"=w321, "error in (no error)"=w316, "Number Steps"=w319, "ListBox"=w313) -> ("error out"=w323:errorcluster)  [unwired: 4 in]
            n157 = local write "Reverse Current Multiplier"(w312) -> ()
            n158 = Number To Decimal String(number=w319) -> (decimal integer string=w326:string)  [unwired: 1 in]
            n159 = Bundle By Name(cluster=w324, "Data Type"=Data_Types."I32", "Name"="HMI_Rect3_4_NumSteps", "Value"=w326) -> (w330:T1)
            n160 = Flatten To String(anything=w330) -> (data string=w329:string)  [unwired: 3 in, 2 out]
            n161 = call <vilib>:"Send Local Message.vi"("message queue in"=w325, "message name"="Write_Tag", "message value"=w329, "error in"=w323) -> ("message queue out"=w328:T5, "error out"=w322:errorcluster)  [unwired: 9 in, 1 out]
            n162 = call <vilib>:"Send Local Message.vi"("message queue in"=w328, "message name"="UpdatePlatingMinutes", "message value"=w326, "error in"=w322) -> ("error out"=w310:errorcluster)  [unwired: 9 in, 2 out]
          }
          frame True {
          }
        }
      }
      frame "EZRecipe" {
        w347 = T7 7 items=["User Home"=0, "User Desktop"=1, "User Documents"=2, "User Application Data"=3, "User Preferences"=4, "User Temporary"=5, "Public Documents"=6, "Public Application Data"=7, "Public Preferences"=8, "Public Cache"=13, "System Core Libraries"=9, "System Installed Libraries"=10, "Application Files"=11, "Boot Volume Root"=12] ("system directory type")
        n163 = local read "Loaded Recipe"() -> (w342:string)
        n164 = call <vilib>:"Get System Directory.vi"("system directory type"=w347) -> ("system directory"=w346:path)  [unwired: 10 in]
        n165 = Build Path(base path=w346, name or relative path="TDK\\CDL0100") -> (appended path=w344:path)
        n166 = control-ref of="Rectifer Settings"() -> (w338:refnum<vi>)
        n167 = Build Path(base path=w344, name or relative path=w342) -> (appended path=w343:path)
        n168 = call "CDL0100 Recipe Creator v1.1.vi"("Previous Recipe Path"=w343) -> ("New Recipe Path"=w339:path, "canceled?"=w335:bool)  [unwired: 1 out]
        n169 = case shown="False" w335 {
          tunnel: w341 -> [w353 w372]
          tunnel: [w348 w372] -> w336
          tunnel: w340 -> [w363 _]
          tunnel: w337 -> [w362 _]
          tunnel: w339 -> [w352 _]
          tunnel: w338 -> [w351 _]
          frame False {
            n170 = call "Read Rectifier Recipe.vi"("selected path"=w352, "error in"=w353) -> ("Left Amps"=w359:dbl[], "Left AmpMins"=w358:dbl[], "Num Steps"=w357:i32, "name"=w349:string, "Rev Mult"=w350:dbl, "Right Amps"=w356:dbl[], "Right AmpMins"=w355:dbl[], "error out"=w354:errorcluster)  [unwired: 5 in, 1 out]
            n171 = local write "Loaded Recipe"(w349) -> ()
            n172 = call "Write Pulse Rectifier Recipe to ListBox.vi"("Right AmpMins"=w355, "Left AmpMins"=w358, "Right Amps"=w356, "Left Amps"=w359, "error in (no error)"=w354, "Number Steps"=w357, "ListBox"=w351) -> ("error out"=w361:errorcluster)  [unwired: 4 in]
            n173 = local write "Reverse Current Multiplier"(w350) -> ()
            n174 = Number To Decimal String(number=w357) -> (decimal integer string=w364:string)  [unwired: 1 in]
            n175 = Bundle By Name(cluster=w362, "Data Type"=Data_Types."I32", "Name"="HMI_Rect3_4_NumSteps", "Value"=w364) -> (w368:T1)
            n176 = Flatten To String(anything=w368) -> (data string=w367:string)  [unwired: 3 in, 2 out]
            n177 = call <vilib>:"Send Local Message.vi"("message queue in"=w363, "message name"="Write_Tag", "message value"=w367, "error in"=w361) -> ("message queue out"=w366:T5, "error out"=w360:errorcluster)  [unwired: 9 in, 1 out]
            n178 = call <vilib>:"Send Local Message.vi"("message queue in"=w366, "message name"="UpdatePlatingMinutes", "message value"=w364, "error in"=w360) -> ("error out"=w348:errorcluster)  [unwired: 9 in, 2 out]
          }
          frame True {
          }
        }
      }
    }
  }
  n179 = while "Message Generator - User Interface Event Handler" {
    tunnel: w20 -> [w374]
    tunnel: w1 -> [w373]
    stop <- w375 stop-if-true
    w376 = 200  # Event Structure Timeout (ms)
    n180 = event shown="[22] \"Settings Button\": Value Change" {
      selector: _ -> [_ _ _ _ _ _ _ _ _ _ _ _ _ _ _ _ _ _ _ _ _ _ _ _ _ _ _ _ _ _ _ _ _ _ _ _ _ _ _ _ _]
      dyn-events: _ -> [_ _ _ _ _ _ _ _ _ _ _ _ _ _ _ _ _ _ _ _ _ _ _ _ _ _ _ _ _ _ _ _ _ _ _ _ _ _ _ _ _]
      timeout: w376 -> [_ _ _ _ _ _ _ _ _ _ _ _ _ _ _ _ _ _ _ _ _ _ _ _ _ _ _ _ _ _ _ _ _ _ _ _ _ _ _ _ _]
      tunnel: [w377 w387 _ TRUE ("Discard?") TRUE ("Discard?") TRUE ("Discard?") TRUE ("Discard?") TRUE ("Discard?") TRUE ("Discard?") TRUE ("Discard?") TRUE ("Discard?") TRUE ("Discard?") TRUE ("Discard?") TRUE ("Discard?") TRUE ("Discard?") TRUE ("Discard?") TRUE ("Discard?") TRUE ("Discard?") TRUE ("Discard?") TRUE ("Discard?") TRUE ("Discard?") FALSE ("Discard?") _ FALSE ("Discard?") FALSE ("Discard?") FALSE ("Discard?") FALSE ("Discard?") FALSE ("Discard?") FALSE ("Discard?") FALSE ("Discard?") FALSE ("Discard?") FALSE ("Discard?") FALSE ("Discard?") FALSE ("Discard?") FALSE ("Discard?") FALSE ("Discard?") _ _ _ _ _] -> w375
      tunnel: w374 -> [w378 w385 _ w394 w398 w402 w406 w410 w414 w418 w422 w426 w430 w434 w438 w442 w446 w450 w454 w458 w462 w468 w471 w475 w480 w493 w504 w515 w526 w530 w544 w564 w574 w584 w594 w606 w608 w610 w615 w637 _]
      tunnel: w373 -> [_ _ _ _ _ _ _ _ _ _ _ _ _ _ _ _ _ _ _ _ _ _ _ _ _ w490 w501 w512 w523 w529 w543 w563 w573 w583 w593 w605 _ _ w616 _ _]
      event Timeout {
        n181 = event-data() -> ()  [unwired: 2 out]
        n182 = call "CheckForAutoLogout.vi"() -> ("Boolean"=w379:bool)  [unwired: 11 in]
        n183 = case shown="True" w379 {
          tunnel: [FALSE ("Discard?") TRUE ("Discard?")] -> w377
          tunnel: w378 -> [_ w381]
          frame False {
          }
          frame True {
            n184 = call <userlib>:"HNE Page Manager (Set).vi"("Next Page"="Home") -> ()  [unwired: 4 in, 1 out]
            n185 = call <vilib>:"Send Local Message.vi"("message queue in"=w381, "message name"="Exit") -> ()  [unwired: 11 in, 3 out]
          }
        }
      }
      event Panel Close? {
        w387 = TRUE ("Discard?")
        # "Intercepts the upper right close panel\noperation to allow a smooth shutdown\nas opposed to immediately killing the app."
        n186 = event-data() -> ()  [unwired: 2 out]
        n187 = call <vilib>:"Send Local Message.vi"("message queue in"=w385, "message name"="Exit") -> ()  [unwired: 11 in, 3 out]
        n188 = event-data("Discard?"=w387) -> ()  [unwired: 1 in, 1 out]
      }
      event Mouse Down? {
        n189 = event-data() -> ("Button"=w391:u16, "Mods"=w390:cluster{"Double Click":bool, "Menu Key":bool}, "PlatMods"=w389:T8)  [unwired: 6 out]
        n190 = Get Date/Time In Seconds() -> (seconds since 1Jan1904=w388:timestamp)
        n191 = shared-variable ".\\Local Variables.lvlib\\LastLogonTime"(w388) -> ()  [unwired: 1 in, 1 out]
        n192 = event-data("Button"=w391, "Mods"=w390, "PlatMods"=w389, "Discard?"=FALSE) -> ()  [unwired: 1 in, 1 out]
      }
      event "Machine": Value Change {
        # "Exit the application\n>> Stop this message generator loop"
        n193 = event-data() -> ()  [unwired: 2 out]
        n194 = call <vilib>:"Send Local Message.vi"("message queue in"=w394, "message name"="Exit") -> ()  [unwired: 11 in, 3 out]
        n195 = call <userlib>:"HNE Page Manager (Set).vi"("Next Page"="Home") -> ()  [unwired: 4 in, 1 out]
      }
      event "Basement 1": Value Change {
        # "Exit the application\n>> Stop this message generator loop"
        n196 = event-data() -> ()  [unwired: 2 out]
        n197 = call <vilib>:"Send Local Message.vi"("message queue in"=w398, "message name"="Exit") -> ()  [unwired: 11 in, 3 out]
        n198 = call <userlib>:"HNE Page Manager (Set).vi"("Next Page"="Basement1") -> ()  [unwired: 4 in, 1 out]
      }
      event "Basement 2": Value Change {
        # "Exit the application\n>> Stop this message generator loop"
        n199 = event-data() -> ()  [unwired: 2 out]
        n200 = call <vilib>:"Send Local Message.vi"("message queue in"=w402, "message name"="Exit") -> ()  [unwired: 11 in, 3 out]
        n201 = call <userlib>:"HNE Page Manager (Set).vi"("Next Page"="Basement2") -> ()  [unwired: 4 in, 1 out]
      }
      event "Basement 3": Value Change {
        # "Exit the application\n>> Stop this message generator loop"
        n202 = event-data() -> ()  [unwired: 2 out]
        n203 = call <vilib>:"Send Local Message.vi"("message queue in"=w406, "message name"="Exit") -> ()  [unwired: 11 in, 3 out]
        n204 = call <userlib>:"HNE Page Manager (Set).vi"("Next Page"="Basement3") -> ()  [unwired: 4 in, 1 out]
      }
      event "Basement 4": Value Change {
        # "Exit the application\n>> Stop this message generator loop"
        n205 = event-data() -> ()  [unwired: 2 out]
        n206 = call <vilib>:"Send Local Message.vi"("message queue in"=w410, "message name"="Exit") -> ()  [unwired: 11 in, 3 out]
        n207 = call <userlib>:"HNE Page Manager (Set).vi"("Next Page"="Basement4") -> ()  [unwired: 4 in, 1 out]
      }
      event "Plater 1": Value Change {
        # "Exit the application\n>> Stop this message generator loop"
        n208 = event-data() -> ()  [unwired: 2 out]
        n209 = call <vilib>:"Send Local Message.vi"("message queue in"=w414, "message name"="Exit") -> ()  [unwired: 11 in, 3 out]
        n210 = call <userlib>:"HNE Page Manager (Set).vi"("Next Page"="Plater1") -> ()  [unwired: 4 in, 1 out]
      }
      event "Plater 3": Value Change {
        # "Exit the application\n>> Stop this message generator loop"
        n211 = event-data() -> ()  [unwired: 2 out]
        n212 = call <vilib>:"Send Local Message.vi"("message queue in"=w418, "message name"="Exit") -> ()  [unwired: 11 in, 3 out]
        n213 = call <userlib>:"HNE Page Manager (Set).vi"("Next Page"="Plater3") -> ()  [unwired: 4 in, 1 out]
      }
      event "Plater 4": Value Change {
        # "Exit the application\n>> Stop this message generator loop"
        n214 = event-data() -> ()  [unwired: 2 out]
        n215 = call <vilib>:"Send Local Message.vi"("message queue in"=w422, "message name"="Exit") -> ()  [unwired: 11 in, 3 out]
        n216 = call <userlib>:"HNE Page Manager (Set).vi"("Next Page"="Plater4") -> ()  [unwired: 4 in, 1 out]
      }
      event "Plater 5": Value Change {
        # "Exit the application\n>> Stop this message generator loop"
        n217 = event-data() -> ()  [unwired: 2 out]
        n218 = call <vilib>:"Send Local Message.vi"("message queue in"=w426, "message name"="Exit") -> ()  [unwired: 11 in, 3 out]
        n219 = call <userlib>:"HNE Page Manager (Set).vi"("Next Page"="Plater5") -> ()  [unwired: 4 in, 1 out]
      }
      event "Plater 6": Value Change {
        # "Exit the application\n>> Stop this message generator loop"
        n220 = event-data() -> ()  [unwired: 2 out]
        n221 = call <vilib>:"Send Local Message.vi"("message queue in"=w430, "message name"="Exit") -> ()  [unwired: 11 in, 3 out]
        n222 = call <userlib>:"HNE Page Manager (Set).vi"("Next Page"="Plater6") -> ()  [unwired: 4 in, 1 out]
      }
      event "Rinse 2": Value Change {
        # "Exit the application\n>> Stop this message generator loop"
        n223 = event-data() -> ()  [unwired: 2 out]
        n224 = call <vilib>:"Send Local Message.vi"("message queue in"=w434, "message name"="Exit") -> ()  [unwired: 11 in, 3 out]
        n225 = call <userlib>:"HNE Page Manager (Set).vi"("Next Page"="Rinse2") -> ()  [unwired: 4 in, 1 out]
      }
      event "Rinse 1": Value Change {
        # "Exit the application\n>> Stop this message generator loop"
        n226 = event-data() -> ()  [unwired: 2 out]
        n227 = call <vilib>:"Send Local Message.vi"("message queue in"=w438, "message name"="Exit") -> ()  [unwired: 11 in, 3 out]
        n228 = call <userlib>:"HNE Page Manager (Set).vi"("Next Page"="Rinse1") -> ()  [unwired: 4 in, 1 out]
      }
      event "Rinse 3": Value Change {
        # "Exit the application\n>> Stop this message generator loop"
        n229 = event-data() -> ()  [unwired: 2 out]
        n230 = call <vilib>:"Send Local Message.vi"("message queue in"=w442, "message name"="Exit") -> ()  [unwired: 11 in, 3 out]
        n231 = call <userlib>:"HNE Page Manager (Set).vi"("Next Page"="Rinse3") -> ()  [unwired: 4 in, 1 out]
      }
      event "Rinse 4": Value Change {
        # "Exit the application\n>> Stop this message generator loop"
        n232 = event-data() -> ()  [unwired: 2 out]
        n233 = call <vilib>:"Send Local Message.vi"("message queue in"=w446, "message name"="Exit") -> ()  [unwired: 11 in, 3 out]
        n234 = call <userlib>:"HNE Page Manager (Set).vi"("Next Page"="Rinse4") -> ()  [unwired: 4 in, 1 out]
      }
      event "Dryer": Value Change {
        # "Exit the application\n>> Stop this message generator loop"
        n235 = event-data() -> ()  [unwired: 2 out]
        n236 = call <vilib>:"Send Local Message.vi"("message queue in"=w450, "message name"="Exit") -> ()  [unwired: 11 in, 3 out]
        n237 = call <userlib>:"HNE Page Manager (Set).vi"("Next Page"="Dryer") -> ()  [unwired: 4 in, 1 out]
      }
      event "Predip": Value Change {
        # "Exit the application\n>> Stop this message generator loop"
        n238 = event-data() -> ()  [unwired: 2 out]
        n239 = call <vilib>:"Send Local Message.vi"("message queue in"=w454, "message name"="Exit") -> ()  [unwired: 11 in, 3 out]
        n240 = call <userlib>:"HNE Page Manager (Set).vi"("Next Page"="Predip") -> ()  [unwired: 4 in, 1 out]
      }
      event "Cleaner": Value Change {
        # "Exit the application\n>> Stop this message generator loop"
        n241 = event-data() -> ()  [unwired: 2 out]
        n242 = call <vilib>:"Send Local Message.vi"("message queue in"=w458, "message name"="Exit") -> ()  [unwired: 11 in, 3 out]
        n243 = call <userlib>:"HNE Page Manager (Set).vi"("Next Page"="Clean") -> ()  [unwired: 4 in, 1 out]
      }
      event "Etch": Value Change {
        # "Exit the application\n>> Stop this message generator loop"
        n244 = event-data() -> ()  [unwired: 2 out]
        n245 = call <vilib>:"Send Local Message.vi"("message queue in"=w462, "message name"="Exit") -> ()  [unwired: 11 in, 3 out]
        n246 = call <userlib>:"HNE Page Manager (Set).vi"("Next Page"="Etch") -> ()  [unwired: 4 in, 1 out]
      }
      event "Enable Plating Cell": Value Change {
        n247 = event-data() -> ("NewVal"=w466:bool)  [unwired: 1 out]
        n248 = call "Validate Plate Tank Enable.vi"("Valve No."=131, "Test Value"=w466, "Tag"="HMI_Tank2_Enable", "Queue in"=w468) -> ()  [unwired: 8 in]
      }
      event "Settings Button": Value Change {
        n249 = event-data() -> ("NewVal"=w470:bool)  [unwired: 6 out]
        n250 = case shown="True" w470 {
          tunnel: w471 -> [_ w472]
          frame False {
          }
          frame True {
            n251 = call <vilib>:"Send Local Message.vi"("message queue in"=w472, "message name"="EZRecipe") -> ()  [unwired: 11 in, 3 out]
          }
        }
      }
      event "Save this Recipe": Value Change {
        n252 = event-data() -> ("NewVal"=w474:bool)  [unwired: 1 out]
        n253 = case shown="True" w474 {
          tunnel: w475 -> [_ w478]
          frame False {
          }
          frame True {
            n254 = call <vilib>:"Send Local Message.vi"("message queue in"=w478, "message name"="Save_Recipe") -> ()  [unwired: 11 in, 3 out]
          }
        }
      }
      event "Load A Recipe": Value Change {
        n255 = event-data() -> ("NewVal"=w479:bool)  [unwired: 1 out]
        n256 = case shown="True" w479 {
          tunnel: w480 -> [_ w483]
          frame False {
          }
          frame True {
            n257 = call <vilib>:"Send Local Message.vi"("message queue in"=w483, "message name"="Load_A_Recipe") -> ()  [unwired: 11 in, 3 out]
          }
        }
      }
      event "Full Drain Plating Cell": Value Change {
        n258 = event-data() -> ("NewVal"=w492:bool)  [unwired: 1 out]
        n259 = Boolean To (0,1)(Boolean=w492) -> (0, 1=w491:i16)
        n260 = Number To Decimal String(number=w491) -> (decimal integer string=w487:string)  [unwired: 1 in]
        n261 = Bundle By Name(cluster=w490, "Data Type"=Data_Types."Boolean", "Name"="HMI_Tank2_Drain", "Value"=w487) -> (w486:T1)
        n262 = Flatten To String(anything=w486) -> (data string=w485:string)  [unwired: 3 in, 2 out]
        n263 = call <vilib>:"Send Local Message.vi"("message queue in"=w493, "message name"="Write_Tag", "message value"=w485) -> ()  [unwired: 10 in, 3 out]
      }
      event "Enable Eductor Motion": Value Change {
        n264 = event-data() -> ("NewVal"=w503:bool)  [unwired: 1 out]
        n265 = Boolean To (0,1)(Boolean=w503) -> (0, 1=w502:i16)
        n266 = Number To Decimal String(number=w502) -> (decimal integer string=w498:string)  [unwired: 1 in]
        n267 = Bundle By Name(cluster=w501, "Data Type"=Data_Types."Boolean", "Name"="HMI_Tank2_Eductor_Motors_Run", "Value"=w498) -> (w497:T1)
        n268 = Flatten To String(anything=w497) -> (data string=w496:string)  [unwired: 3 in, 2 out]
        n269 = call <vilib>:"Send Local Message.vi"("message queue in"=w504, "message name"="Write_Tag", "message value"=w496) -> ()  [unwired: 10 in, 3 out]
      }
      event "Enable Rack Motion": Value Change {
        n270 = event-data() -> ("NewVal"=w514:bool)  [unwired: 1 out]
        n271 = Boolean To (0,1)(Boolean=w514) -> (0, 1=w513:i16)
        n272 = Number To Decimal String(number=w513) -> (decimal integer string=w509:string)  [unwired: 1 in]
        n273 = Bundle By Name(cluster=w512, "Data Type"=Data_Types."Boolean", "Name"="HMI_Tank2_Rack_Motor_Run", "Value"=w509) -> (w508:T1)
        n274 = Flatten To String(anything=w508) -> (data string=w507:string)  [unwired: 3 in, 2 out]
        n275 = call <vilib>:"Send Local Message.vi"("message queue in"=w515, "message name"="Write_Tag", "message value"=w507) -> ()  [unwired: 10 in, 3 out]
      }
      event "Enable Suck Pump": Value Change {
        n276 = event-data() -> ("NewVal"=w525:bool)  [unwired: 1 out]
        n277 = Boolean To (0,1)(Boolean=w525) -> (0, 1=w524:i16)
        n278 = Number To Decimal String(number=w524) -> (decimal integer string=w520:string)  [unwired: 1 in]
        n279 = Bundle By Name(cluster=w523, "Data Type"=Data_Types."Boolean", "Name"="HMI_Tnk2_Enable_SuckPump", "Value"=w520) -> (w519:T1)
        n280 = Flatten To String(anything=w519) -> (data string=w518:string)  [unwired: 3 in, 2 out]
        n281 = call <vilib>:"Send Local Message.vi"("message queue in"=w526, "message name"="Write_Tag", "message value"=w518) -> ()  [unwired: 10 in, 3 out]
      }
      event "Start Cycle": Value Change {
        n282 = event-data() -> ("NewVal"=w528:bool)  [unwired: 1 out]
        n283 = case shown="True" w528 {
          tunnel: w530 -> [_ w541]
          tunnel: w528 -> [_ w540]
          tunnel: w529 -> [_ w538]
          frame False {
          }
          frame True {
            n284 = Boolean To (0,1)(Boolean=w540) -> (0, 1=w539:i16)
            n285 = Number To Decimal String(number=w539) -> (decimal integer string=w535:string)  [unwired: 1 in]
            n286 = Bundle By Name(cluster=w538, "Data Type"=Data_Types."Boolean", "Name"="HMI_Rect3_4_Cycle", "Value"=w535) -> (w534:T1)
            n287 = Flatten To String(anything=w534) -> (data string=w533:string)  [unwired: 3 in, 2 out]
            n288 = call <vilib>:"Send Local Message.vi"("message queue in"=w541, "message name"="Write_Tag", "message value"=w533) -> ()  [unwired: 10 in, 3 out]
          }
        }
      }
      event "Cancel Cycle": Value Change {
        n289 = event-data() -> ("NewVal"=w542:bool)  [unwired: 1 out]
        n290 = case shown="True" w542 {
          tunnel: w544 -> [_ w555]
          tunnel: w542 -> [_ w554]
          tunnel: w543 -> [_ w552]
          frame False {
          }
          frame True {
            n291 = Boolean To (0,1)(Boolean=w554) -> (0, 1=w553:i16)
            n292 = Number To Decimal String(number=w553) -> (decimal integer string=w549:string)  [unwired: 1 in]
            n293 = Bundle By Name(cluster=w552, "Data Type"=Data_Types."Boolean", "Name"="HMI_Rect3_4_CycleStop", "Value"=w549) -> (w548:T1)
            n294 = Flatten To String(anything=w548) -> (data string=w547:string)  [unwired: 3 in, 2 out]
            n295 = call <vilib>:"Send Local Message.vi"("message queue in"=w555, "message name"="Write_Tag", "message value"=w547) -> ()  [unwired: 10 in, 3 out]
          }
        }
      }
      event "Eductor RPM": Value Change {
        # "Uaes Tank 1 Freq source"
        n296 = event-data() -> ("NewVal"=w557:dbl)  [unwired: 1 out]
        n297 = Number To Fractional String(number=w557) -> (F-format string=w556:string)  [unwired: 3 in]
        n298 = Bundle By Name(cluster=w563, "Data Type"=Data_Types."Double", "Name"="HMI_Tnk1_Eductor_RPM", "Value"=w556) -> (w560:T1)
        n299 = Flatten To String(anything=w560) -> (data string=w559:string)  [unwired: 3 in, 2 out]
        n300 = call <vilib>:"Send Local Message.vi"("message queue in"=w564, "message name"="Write_Tag", "message value"=w559) -> ()  [unwired: 10 in, 3 out]
      }
      event "Rack RPM": Value Change {
        # "Uses Tank 1 freq source"
        n301 = event-data() -> ("NewVal"=w567:dbl)  [unwired: 1 out]
        n302 = Number To Fractional String(number=w567) -> (F-format string=w566:string)  [unwired: 3 in]
        n303 = Bundle By Name(cluster=w573, "Data Type"=Data_Types."Double", "Name"="HMI_Tnk1_Rack_RPM", "Value"=w566) -> (w570:T1)
        n304 = Flatten To String(anything=w570) -> (data string=w569:string)  [unwired: 3 in, 2 out]
        n305 = call <vilib>:"Send Local Message.vi"("message queue in"=w574, "message name"="Write_Tag", "message value"=w569) -> ()  [unwired: 10 in, 3 out]
      }
      event "Total Inflow (L/min)": Value Change {
        n306 = event-data() -> ("NewVal"=w577:dbl)  [unwired: 1 out]
        n307 = Number To Fractional String(number=w577) -> (F-format string=w576:string)  [unwired: 3 in]
        n308 = Bundle By Name(cluster=w583, "Data Type"=Data_Types."Double", "Name"="HMI_TNK2_Flow_Setpoint", "Value"=w576) -> (w580:T1)
        n309 = Flatten To String(anything=w580) -> (data string=w579:string)  [unwired: 3 in, 2 out]
        n310 = call <vilib>:"Send Local Message.vi"("message queue in"=w584, "message name"="Write_Tag", "message value"=w579) -> ()  [unwired: 10 in, 3 out]
      }
      event "Supply Pressure (kPa)": Value Change {
        n311 = event-data() -> ("NewVal"=w587:dbl)  [unwired: 1 out]
        n312 = Number To Fractional String(number=w587) -> (F-format string=w586:string)  [unwired: 3 in]
        n313 = Bundle By Name(cluster=w593, "Data Type"=Data_Types."Double", "Name"="HMI_BAS_TNK1_P_Setpoint", "Value"=w586) -> (w590:T1)
        n314 = Flatten To String(anything=w590) -> (data string=w589:string)  [unwired: 3 in, 2 out]
        n315 = call <vilib>:"Send Local Message.vi"("message queue in"=w594, "message name"="Write_Tag", "message value"=w589) -> ()  [unwired: 10 in, 3 out]
      }
      event "Suck Pump fraction of inflow": Value Change {
        n316 = event-data() -> ("NewVal"=w597:dbl)  [unwired: 1 out]
        n317 = Divide(x=w597, y=100.0) -> (x/y=w596:dbl)
        n318 = Number To Fractional String(number=w596) -> (F-format string=w599:string)  [unwired: 3 in]
        n319 = Bundle By Name(cluster=w605, "Data Type"=Data_Types."Double", "Name"="HMI_TNK2_SuckPmpFrac_Setpoint", "Value"=w599) -> (w602:T1)
        n320 = Flatten To String(anything=w602) -> (data string=w601:string)  [unwired: 3 in, 2 out]
        n321 = call <vilib>:"Send Local Message.vi"("message queue in"=w606, "message name"="Write_Tag", "message value"=w601) -> ()  [unwired: 10 in, 3 out]
      }
      event Menu Selection (User) {
        # "Add run-time menu items to the message\nqueue. The message handler case names must match the menu ItemTag names."
        n322 = event-data() -> ("ItemTag"=w609:string)  [unwired: 1 out]
        n323 = call <vilib>:"Send Local Message.vi"("message queue in"=w608, "message name"=w609) -> ()  [unwired: 11 in, 3 out]
      }
      event "Cell T Last Hr": Value Change {
        n324 = event-data() -> ("NewVal"=w611:bool)  [unwired: 3 out]
        n325 = case shown="True" w611 {
          tunnel: w610 -> [_ w614]
          frame False {
          }
          frame True {
            n326 = call <vilib>:"Send Local Message.vi"("message queue in"=w614, "message name"="DisplayLastHr", "message value"="TNK2_Temperature") -> ()  [unwired: 10 in, 3 out]
          }
        }
      }
      event "Rectifer Settings": Mouse Down {
        n327 = event-data() -> ("CtlRef"=w621:refnum<vi>, "Coords"=w620:T9, "Button"=w619:u16)  [unwired: 5 out]
        n328 = call "Handle Rectifer Step Selection.vi"("Coords"=w620, "Button"=w619, "MulticolumnListbox in"=w621) -> ("Row"=w617:i32)  [unwired: 8 in]
        n329 = Greater Than 0?(x=w617) -> (x > 0?=w618:bool)
        n330 = case shown="True" w618 {
          tunnel: w617 -> [_ w627]
          tunnel: w616 -> [_ w625]
          tunnel: w615 -> [_ w626]
          frame False {
          }
          frame True {
            n331 = Number To Decimal String(number=w627) -> (decimal integer string=w622:string)  [unwired: 1 in]
            n332 = Bundle By Name(cluster=w625, "Data Type"=Data_Types."I32", "Name"="HMI_Rect3_4_NumSteps", "Value"=w622) -> (w629:T1)
            n333 = Flatten To String(anything=w629) -> (data string=w628:string)  [unwired: 3 in, 2 out]
            n334 = call <vilib>:"Send Local Message.vi"("message queue in"=w626, "message name"="Write_Tag", "message value"=w628) -> ("message queue out"=w624:T5)  [unwired: 10 in, 2 out]
            n335 = call <vilib>:"Send Local Message.vi"("message queue in"=w624, "message name"="UpdatePlatingMinutes", "message value"=w622) -> ()  [unwired: 10 in, 3 out]
          }
        }
      }
      event "Rectifer Settings": Edit Cell {
        n336 = event-data() -> ("CtlRef"=w641:refnum<vi>, "String"=w640:string, "Coords"=w642:T10)  [unwired: 4 out]
        n337 = call "Data Check Rectifier Settings.vi"("String"=w640, "Coords"=w642, "MulticolumnListbox in"=w641) -> ("error out"=w633:errorcluster)  [unwired: 7 in, 1 out]
        n338 = shared-variable-read(refnum<k21> "ni.var.psp://z004551/CDL0100 ReadWriteTags/HMI_Rect3_4_NumSteps" ("shared variable refnum in"), 0) -> (w636:i32)  [unwired: 1 in, 3 out]
        n339 = Number To Decimal String(number=w636) -> (decimal integer string=w635:string)  [unwired: 1 in]
        n340 = call <vilib>:"Send Local Message.vi"("message queue in"=w637, "message name"="UpdatePlatingMinutes", "message value"=w635, "error in"=w633) -> ()  [unwired: 9 in, 3 out]
      }
      event "MO": Value Change {
        n341 = event-data() -> ("NewVal"=w643:string)  [unwired: 6 out]
        n342 = shared-variable ".\\Local Variables.lvlib\\PT2_MO"(w643) -> ()  [unwired: 1 in, 1 out]
      }
    }
  }
  n343 = call-poly <vilib>:"Get Connection Reference.vi"("error in"=w8, "connection info in"=w9) -> ("error out"=w12:errorcluster, "connection ID out"=w11:refnum<k5>)  [unwired: 8 out]
  n344 = TCP Close Connection(connection ID=w11, error in (no error)=w12) -> (error out=w14:errorcluster)  [unwired: 2 out]
  n345 = call <vilib>:"Error to Warning.vi"("1st Error to Convert"=w13, "error in"=w14) -> ("warning out"=w10:errorcluster)  [unwired: 3 in, 10 out]
  n346 = call <vilib>:"Simple Error Handler.vi"("error in (no error)"=w10) -> ()  [unwired: 4 in, 5 out]
